vi "dat_thermistors.vi"(3 "Timeout":i32) -> (15 "FIFO_timeout":bool, 20 "v_pb_1_t":fxp<+/-,24,5>, 21 "v_pb_2_t":fxp<+/-,24,5>, 22 "v_rb_t":fxp<+/-,24,5>, 23 "v_pod_t":fxp<+/-,24,5>, 24 "v_pneum_tank_t":fxp<+/-,24,5>, 25 "v_extra_1_t":fxp<+/-,24,5>, 26 "v_extra_2_t":fxp<+/-,24,5>)   [LabVIEW 2018]
uses:
  <vilib>/rvi/DataTransferAndStorage/Container/Common/niFpgaContainerExecOnDevCompGetState.vi
  <vilib>/rvi/Emulation/niFpgaEmulationIsFPGAContextNoSignature.vi
  <vilib>/rvi/Emulation/niFpgaSctlEmulationGetInTimedLoop.vi
  <vilib>/rvi/errors/niFpgaSetErrorForExecOnDevCompSimple.vi
  <vilib>/rvi/eio/common/nirviEmuReportErrorAndStop.vi
  <vilib>/rvi/DataTransferAndStorage/Container/Common/niFpgaContainerGetUniqueNameForEmu.vi
  <vilib>/rvi/FIFO/Fifo_Resource/nirvififoEmulationSetSize.vi
  <vilib>/rvi/FIFO/Fifo_Resource/nirviFifoEmulationQueueMgr.vi
  <instcachedir>/0/nirviFifoEmulationQueueMgr_E5CAEC123FF24DC58D834DCA3CDAA9B5.lvgen/nirviFifoEmulationQueueMgr_E5CAEC123FF24DC58D834DCA3CDAA9B5_002.vi
  <vilib>/rvi/FIFO/Fifo_Resource/nirvififoEmulationDetermineInputValidOut.vi
  <vilib>/rvi/FIFO/Fifo_Resource/nirvififoEmulationCreateLock.vi
  <vilib>/rvi/Emulation/niFpgaProcessEmulError.vi
  <vilib>/rvi/FIFO/Fifo_Resource/nirvififoEmulationObtainLock.vi
  <vilib>/rvi/FIFO/Fifo_Resource/nirvififoEmulationReleaseLock.vi
  <vilib>/rvi/occurrence/nirviWaitOnOccurrenceBase.vi
  <vilib>/rvi/errors/nirviReportUnexpectedCaseInternalError.vi
  <vilib>/rvi/errors/nirviReportUnexpectedCaseInternalError (U32).vi
  <vilib>/Utility/error.llb/Clear Errors.vi
  <vilib>/rvi/interface/RandomDataEmulation/niFpgaRandomDataHandleErrors.vi
  <vilib>/rvi/DataTransferAndStorage/Container/XNode/niFpgaContainer.xnode
  <vilib>/rvi/FIFO/Fifo_Resource/niFpgaFifoEmulationRefIn.vi
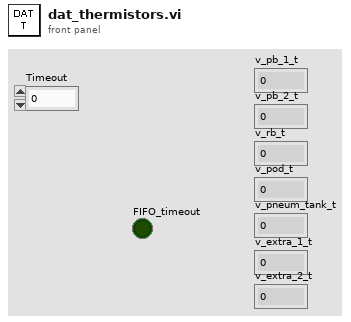
[diagram p1: front panel]
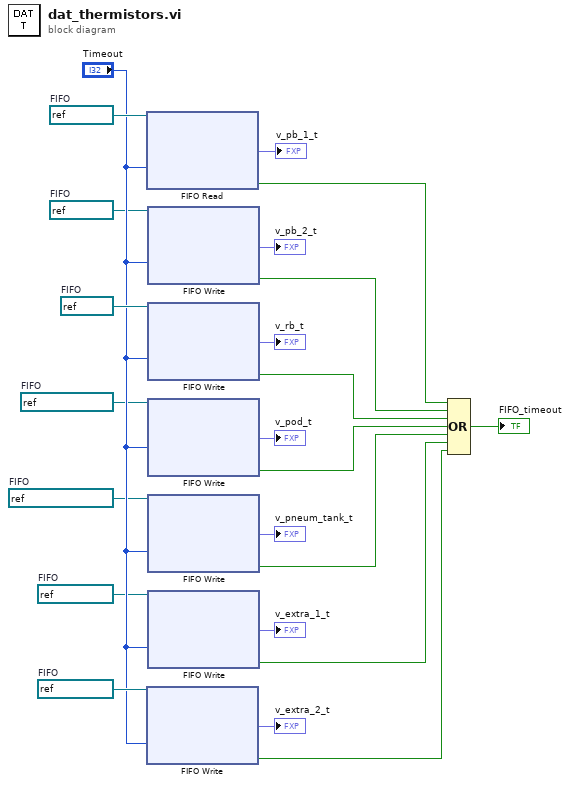
[diagram p0: block diagram]
diagram:
  w10 = refnum<k21> "T_pod_temp"  # FIFO
  w11 = refnum<k21> "T_extra_1"  # FIFO
  w13 = refnum<k21> "T_PB_2"  # FIFO
  w17 = refnum<k21> "T_extra_2"  # FIFO
  w12 = refnum<k21> "T_pneum_tank"  # FIFO
  w22 = refnum<k21> "T_RB"  # FIFO
  w23 = refnum<k21> "T_PB_1"  # FIFO
  n1 = xnode "FIFO Read"("Timeout"="Timeout", "FIFO In"=w23) -> ("Element"=→"v_pb_1_t":fxp<+/-,24,5>, "Timed Out?"=w21:bool)  [unwired: 1 out]
  n2 = xnode "FIFO Write"("Timeout"="Timeout", "FIFO In"=w17) -> ("Element"=→"v_extra_2_t":fxp<+/-,24,5>, "Timed Out?"=w16:bool)  [unwired: 1 out]
  n3 = xnode "FIFO Write"("Timeout"="Timeout", "FIFO In"=w13) -> ("Element"=→"v_pb_2_t":fxp<+/-,24,5>, "Timed Out?"=w20:bool)  [unwired: 1 out]
  n4 = xnode "FIFO Write"("Timeout"="Timeout", "FIFO In"=w22) -> ("Element"=→"v_rb_t":fxp<+/-,24,5>, "Timed Out?"=w4:bool)  [unwired: 1 out]
  n5 = xnode "FIFO Write"("Timeout"="Timeout", "FIFO In"=w10) -> ("Element"=→"v_pod_t":fxp<+/-,24,5>, "Timed Out?"=w3:bool)  [unwired: 1 out]
  n6 = xnode "FIFO Write"("Timeout"="Timeout", "FIFO In"=w12) -> ("Element"=→"v_pneum_tank_t":fxp<+/-,24,5>, "Timed Out?"=w19:bool)  [unwired: 1 out]
  n7 = xnode "FIFO Write"("Timeout"="Timeout", "FIFO In"=w11) -> ("Element"=→"v_extra_1_t":fxp<+/-,24,5>, "Timed Out?"=w15:bool)  [unwired: 1 out]
  n8 = Compound Arithmetic op=OR(w21, w20, w4, w3, w19, w15, w16) -> (→"FIFO_timeout":bool)
